vi "Main.vi"() -> ()   [LabVIEW 2025]
uses:
  Controls/Wheel_data.ctl
  Controls/Spork plot.ctl
  Controls/Spoke_stats.ctl
  Controls/Spork type.ctl
  Controls/Tension.ctl
  Controls/Tension_Output.ctl
  Controls/Runout.ctl
  Controls/Runout Output.ctl
  Controls/Nippel Turn Direction.ctl
  Controls/Aditional Info.ctl
  Controls/States.ctl
  <vilib>/Utility/NIReport.llb/NI_ReportGenerationCore.lvlib
panel:
  in  "Tab Control":enum32{"General", "Runout", "Tencion", "Export"}(tab)
  in  "Spokes":T1 {"Spokes crosses" min=0 max=4; "Spokes number" min=0 max=200 step=2}
  out "Wheel Visualation":cluster{dbl[], dbl[]}[](graph)
  in  "Stop":bool
  in  "Runout":bool
  out "Runout Graph":T3[](graph)
  out "Spork Measured":i32[](array[numeric])
  out "Runout Measurement":T4[](array[typedef])
  out "Runout Standard Diviation":dbl
  out "Runout Average":dbl
  in  "Spoke Tension Left":dbl[](array[numeric])
  in  "Variance":dbl min=0.0 max=25.0 step=5.0 format="%.0f %%"
  in  "Spoke Tension Right":dbl[](array[numeric])
  out "Tension Output Left":T6[](array[typedef])
  out "Tension Output Right":T6[](array[typedef])
  out "Spokes Tension":cluster{dbl[], dbl[]}[](graph)
  out "Average Tencion Right [kgf]":dbl
  out "Standard Diviation Right [kgf]":dbl
  out "Standard Diviation Left [kgf]":dbl
  out "Average Tencion Left [kgf]":dbl
  in  "Aditional Information":T7
  in  "Preview in Broweser":bool
  in  "Print":bool
  in  "Printer":u32(ring) items=["Default", "OneNote (Desktop) - Protected", "OneNote (Desktop)", "Microsoft Print to PDF"]
  in  "Wheel data":T8
  out "error out":errorcluster
  in  "error in":errorcluster
  # "Pass?"
  # "Pass?"
  # "Tension [kgf]"
  # "Tension [kgf]"
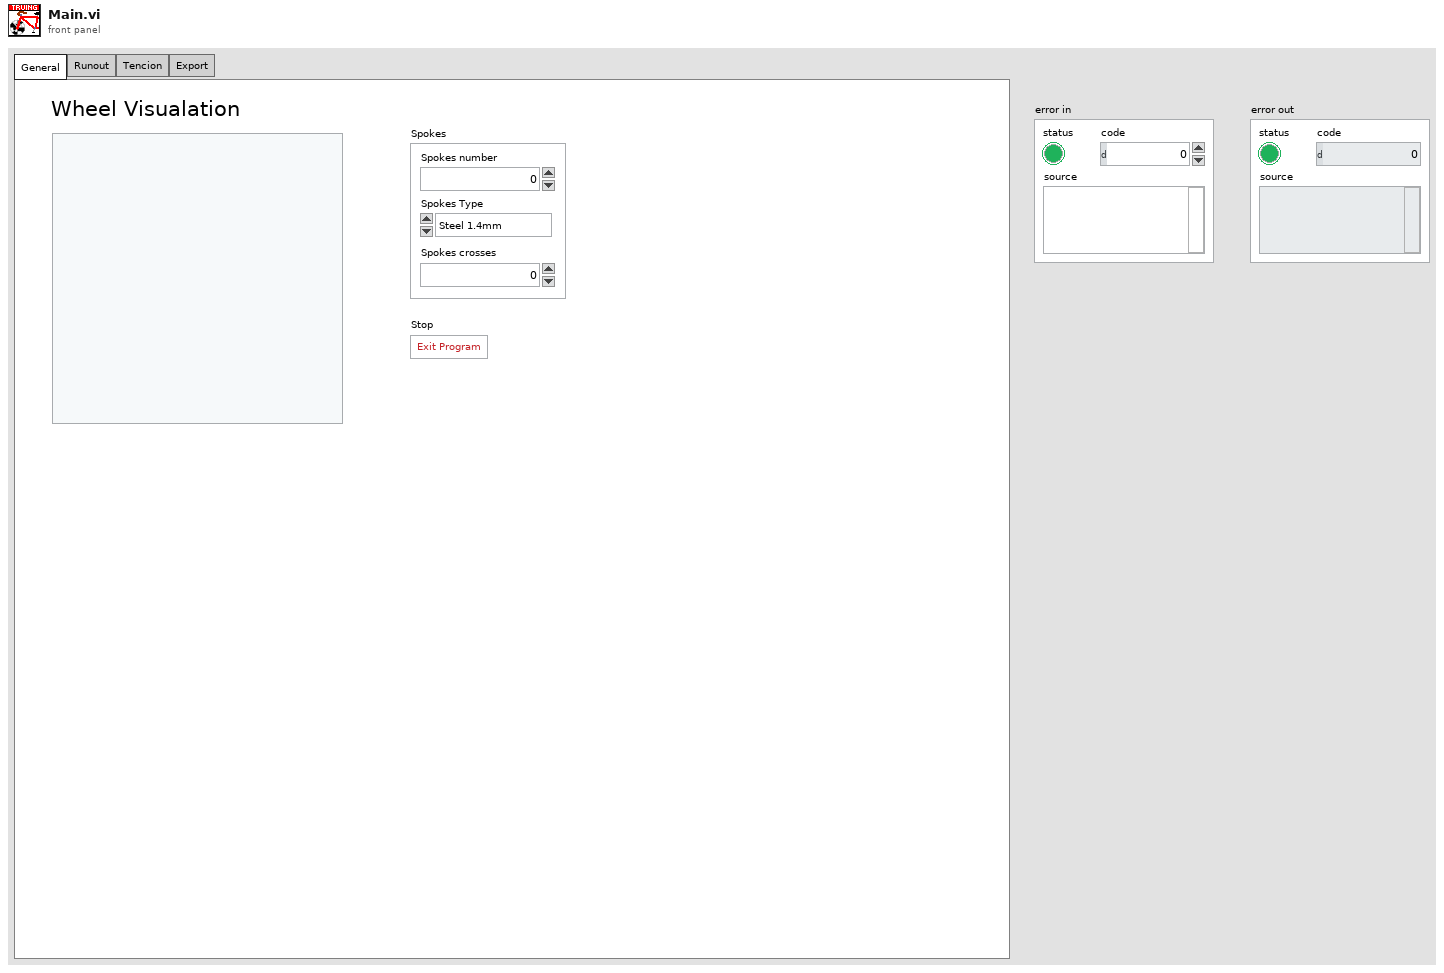
[diagram p1: front panel]
types:
  T1 = typedef "Spoke_stats.ctl" = cluster{"Spokes number":i32, "Spokes crosses":i32, "Spokes Type":T2}
  T2 = typedef "Spork type.ctl" = enum16{"Steel 1.4mm", "Steel 1.5mm", "Steel 1.6mm", "Steel 1.7mm", "Steel 1.8mm", "Steel 2mm", "Steel 2.3mm", "Steel 2.5mm", "Steel 2.6mm", "Aluminum 2.28mm", "Aluminum 2.54mm", "Aluminum 2.8mm", "Aluminum 3.3mm"}
  T3 = typedef "Spork plot.ctl" = cluster{"X":dbl[], "Y":dbl[]}
  T4 = typedef "Runout Output.ctl" = cluster{"Value":dbl, "Nippel Direction":T5}
  T5 = typedef "Nippel Turn Direction.ctl" = u16
  T6 = typedef "Tension_Output.ctl" = cluster{"Tenction [kgf]":dbl, "Within Limit":bool}
  T7 = typedef "Aditional Info.ctl" = cluster{"Name":string, "Rims":string, "Hub":string, "Notes":string, "Spokes":string, "Type":enum32{"Item 0", "Item 1"}, "Mechanic's Name":string}
  T8 = typedef "Wheel_data.ctl" = cluster{"Wheel Grapth":T3[], "Spokes":T1, "Tension":T9, "Runout":T10, "Avaliable Printers":string[], "Aditional Info":T7}
  T9 = typedef "Tension.ctl" = cluster{"Spokes Tension Left":dbl[], "Tension Graph":T3[], "Average Left":dbl, "Variance":dbl, "Std Div Left":dbl, "Average Right":dbl, "Std Div Right":dbl, "Tension Output Left":T6[], "Tension Output Right":T6[], "Spokes Tension Right":dbl[]}
  T10 = typedef "Runout.ctl" = cluster{"Runout Output":T4[], "Runout Graph":T3[], "Average":dbl, "Std Div":dbl, "Spoke Measured":i32[]}
  T11 = typedef "States.ctl" = enum16{"Error", "Init", "Idle", "Draw Wheel", "Tension", "Runout", "Report", "Stop"}
  T12 = typedef "LVStringsAndValuesArrayTypeDef_U32.ctl" = cluster{"String":string, "Value":u32}[]
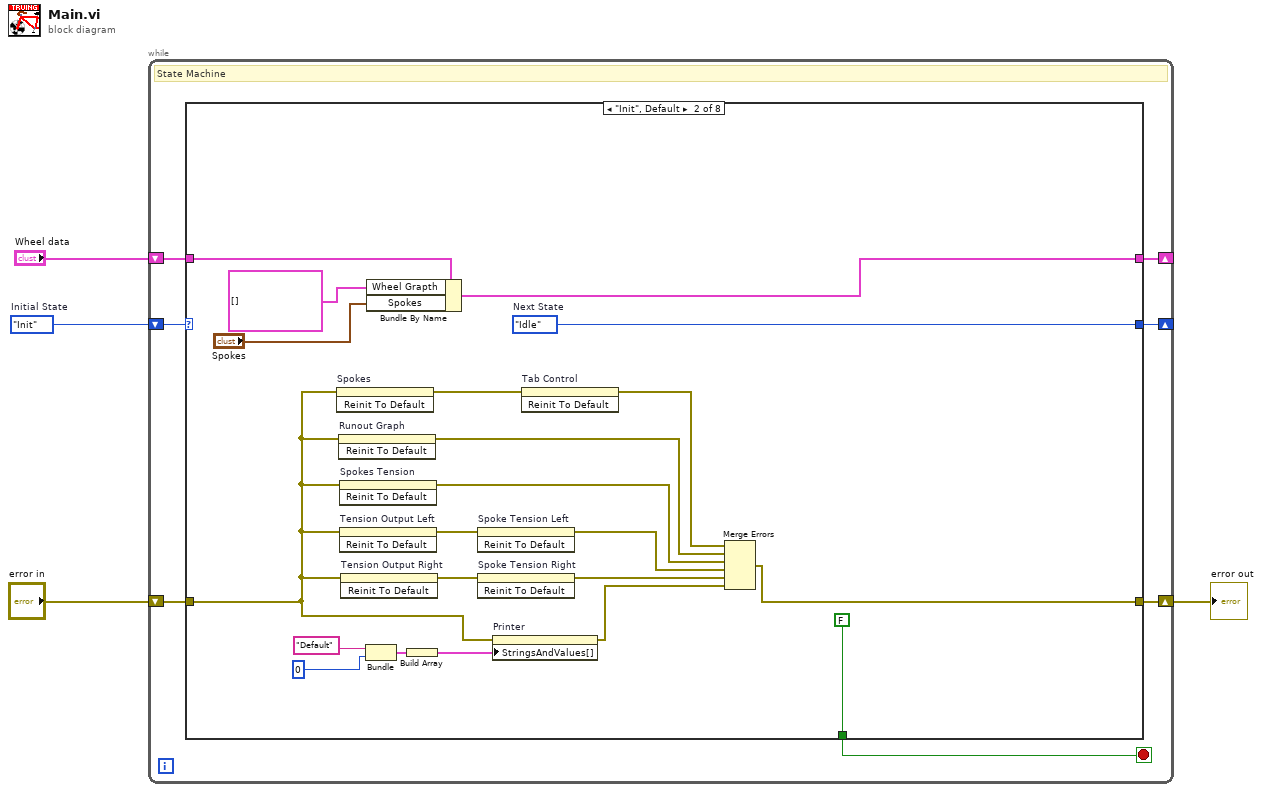
[diagram p0: block diagram]
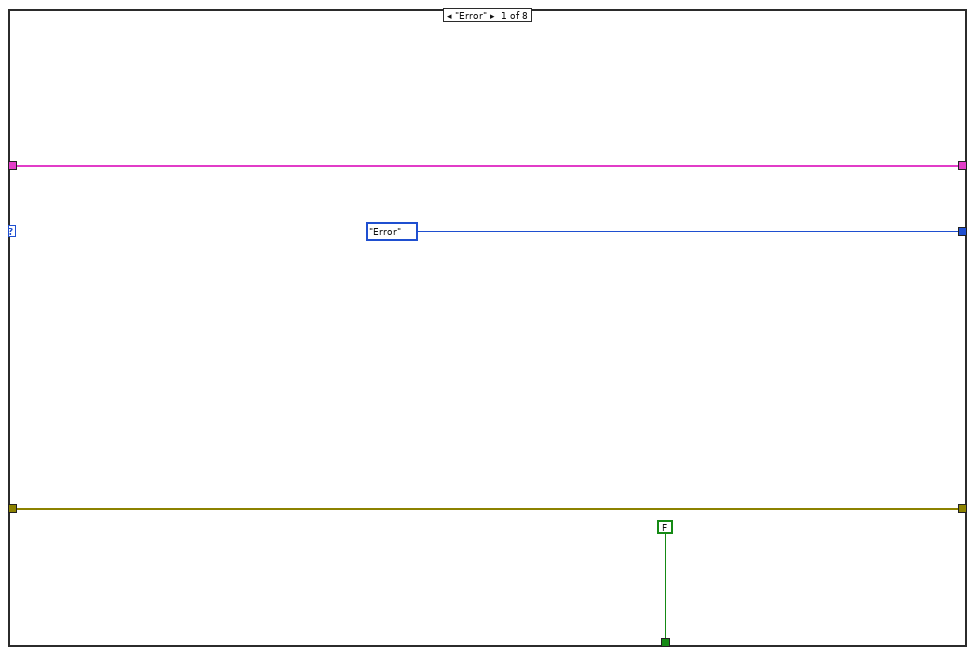
[diagram p2: hidden frame]
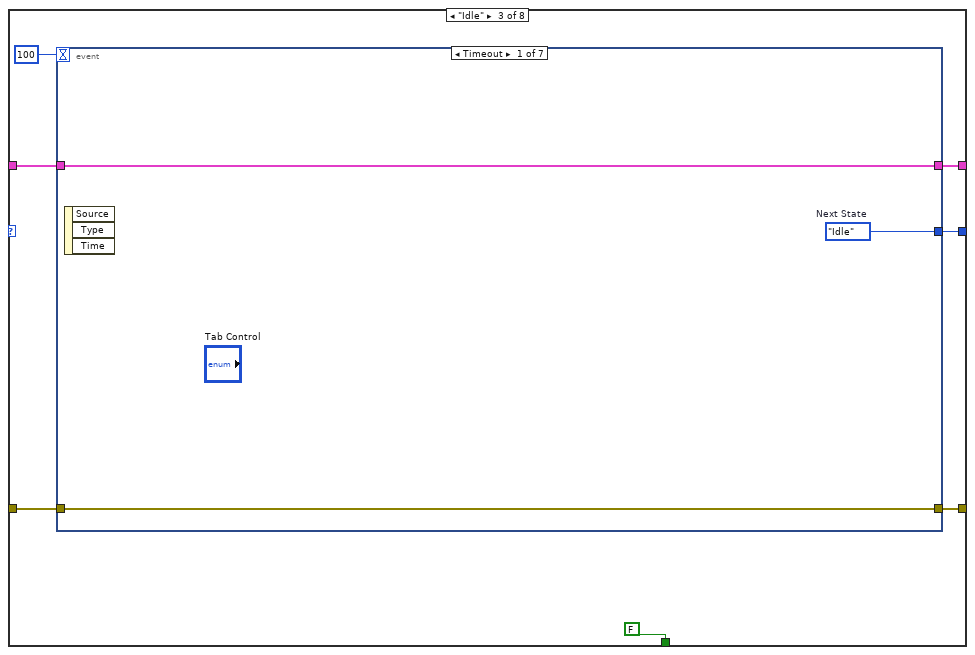
[diagram p3: hidden frame]
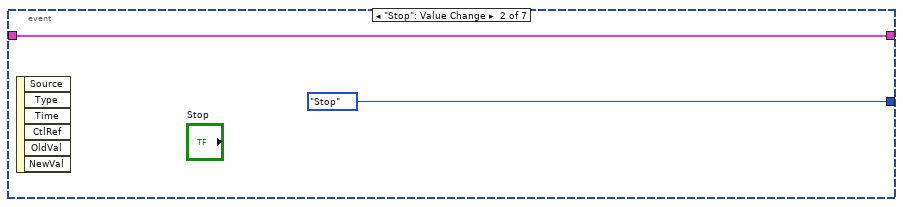
[diagram p4: hidden frame]
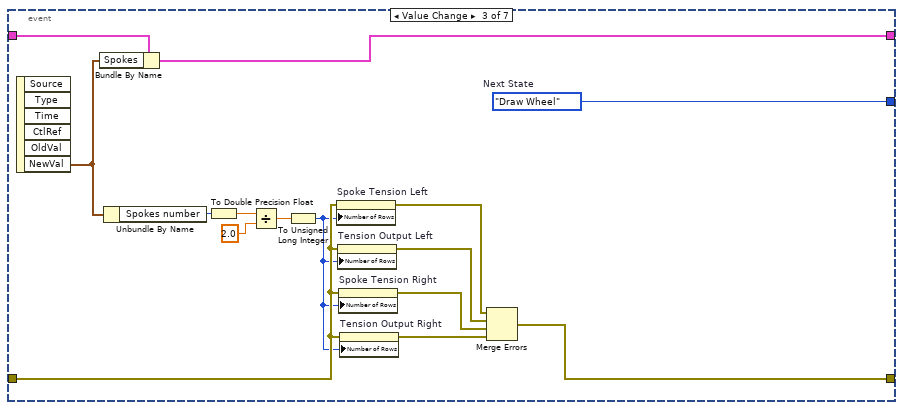
[diagram p5: hidden frame]
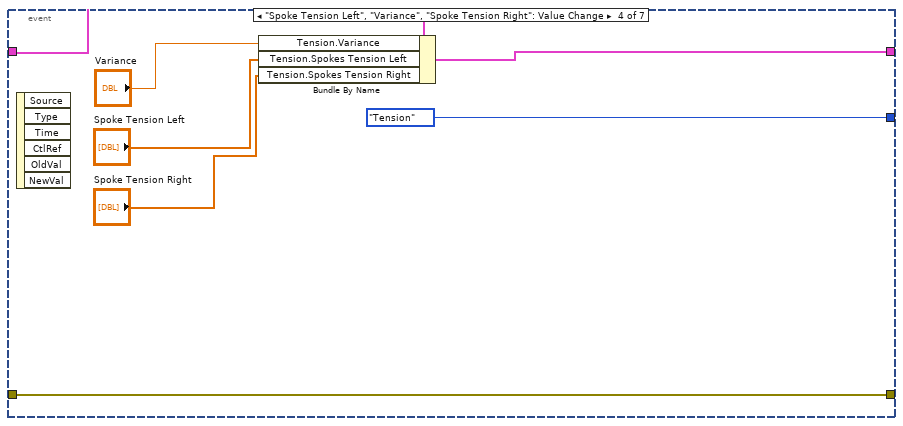
[diagram p6: hidden frame]
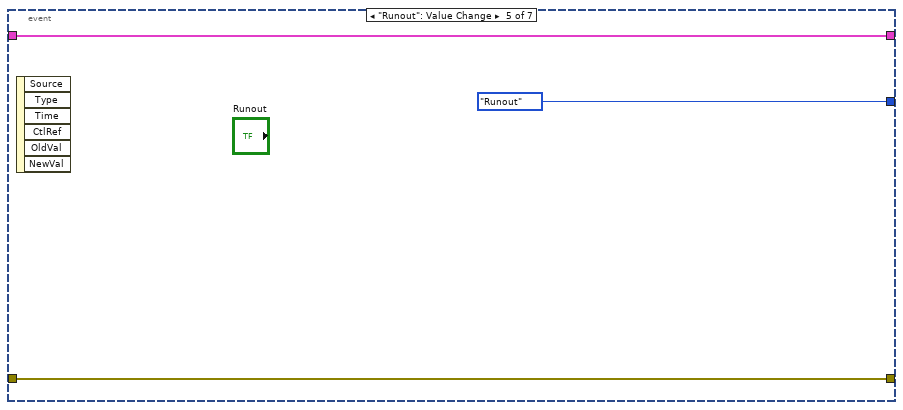
[diagram p7: hidden frame]
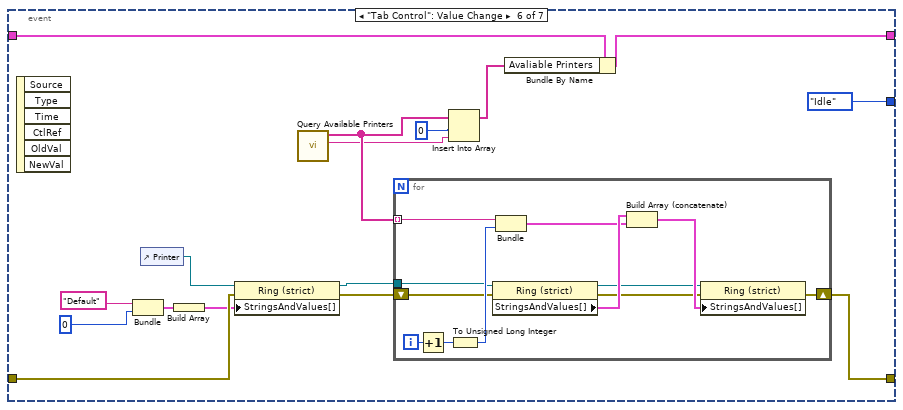
[diagram p8: hidden frame]
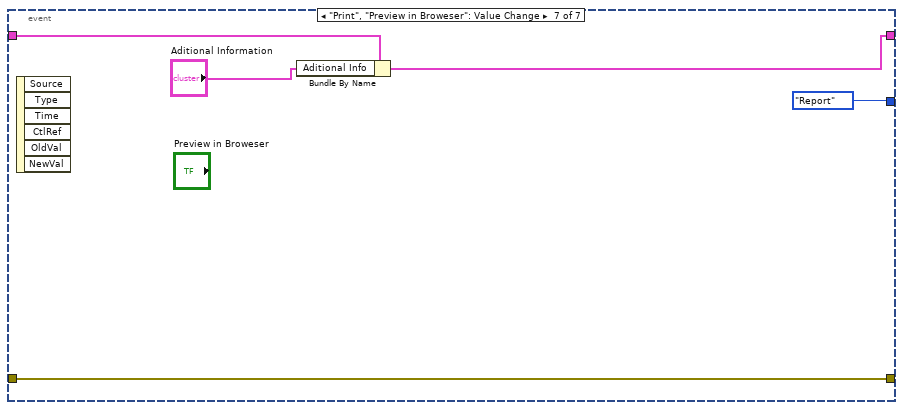
[diagram p9: hidden frame]
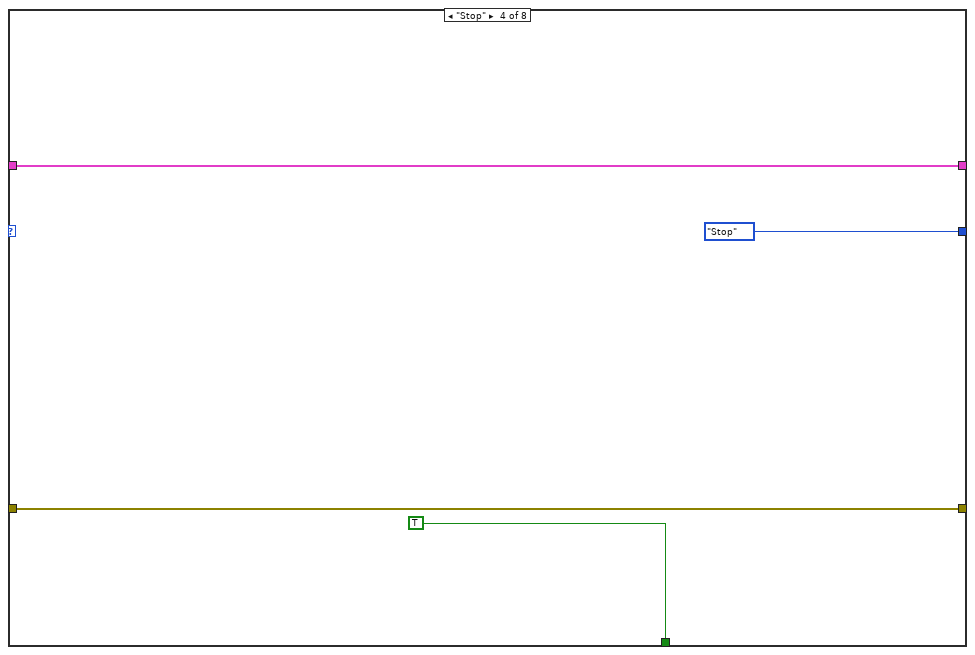
[diagram p10: hidden frame]
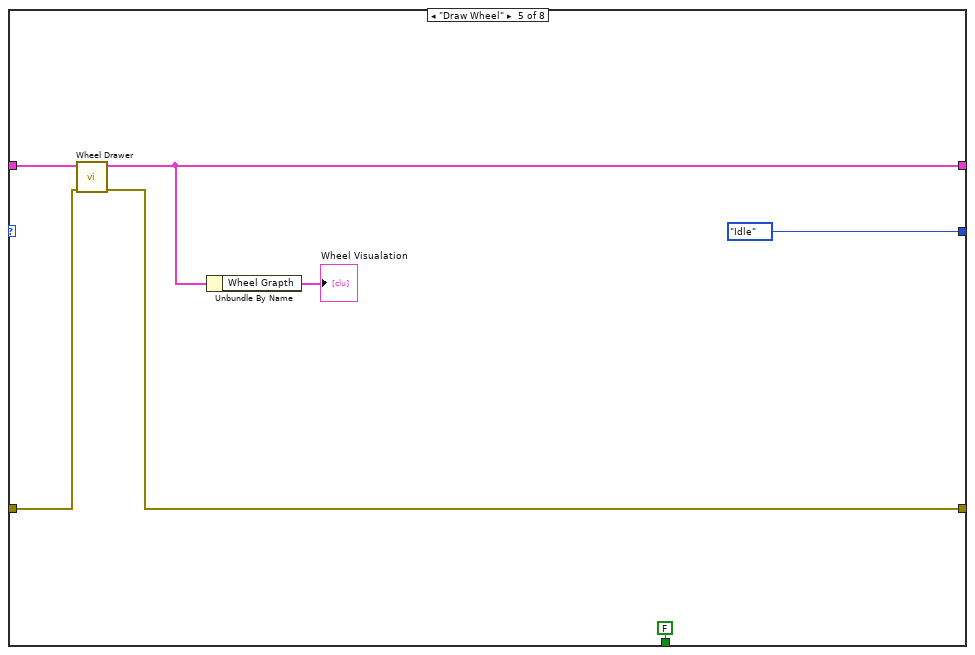
[diagram p11: hidden frame]
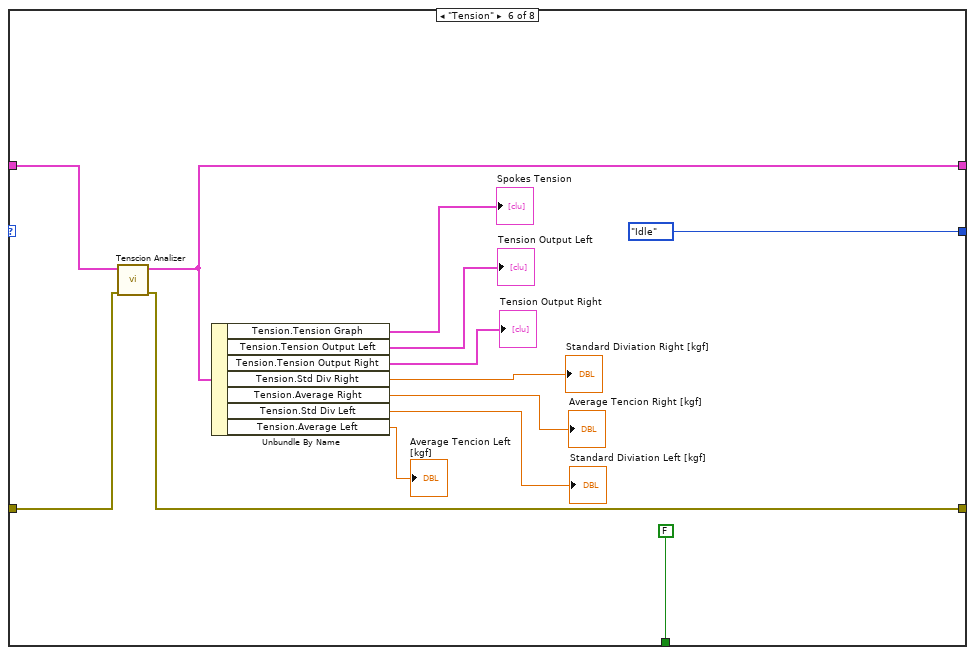
[diagram p12: hidden frame]
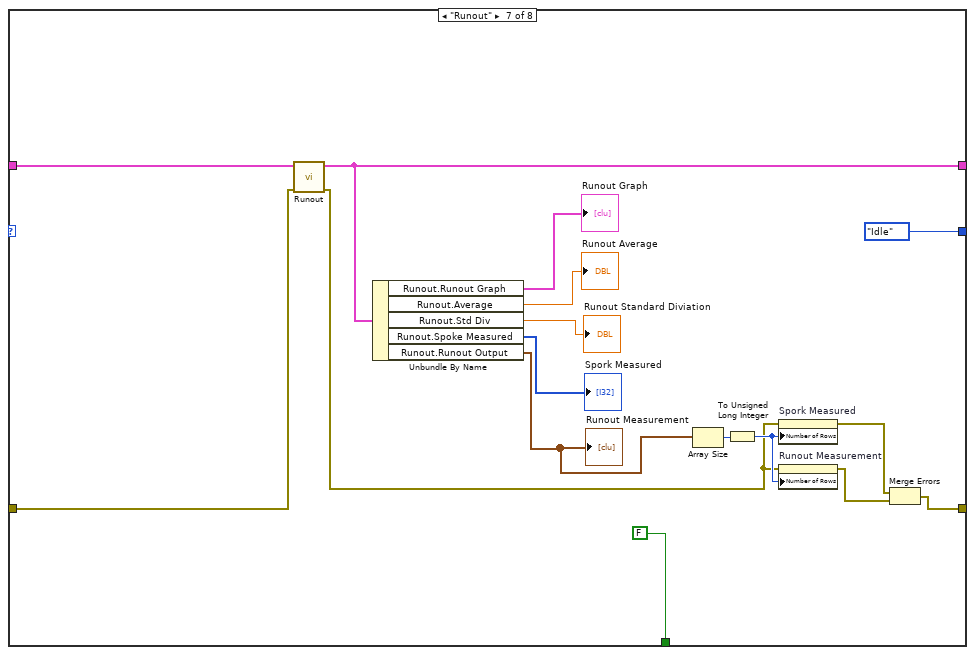
[diagram p13: hidden frame]
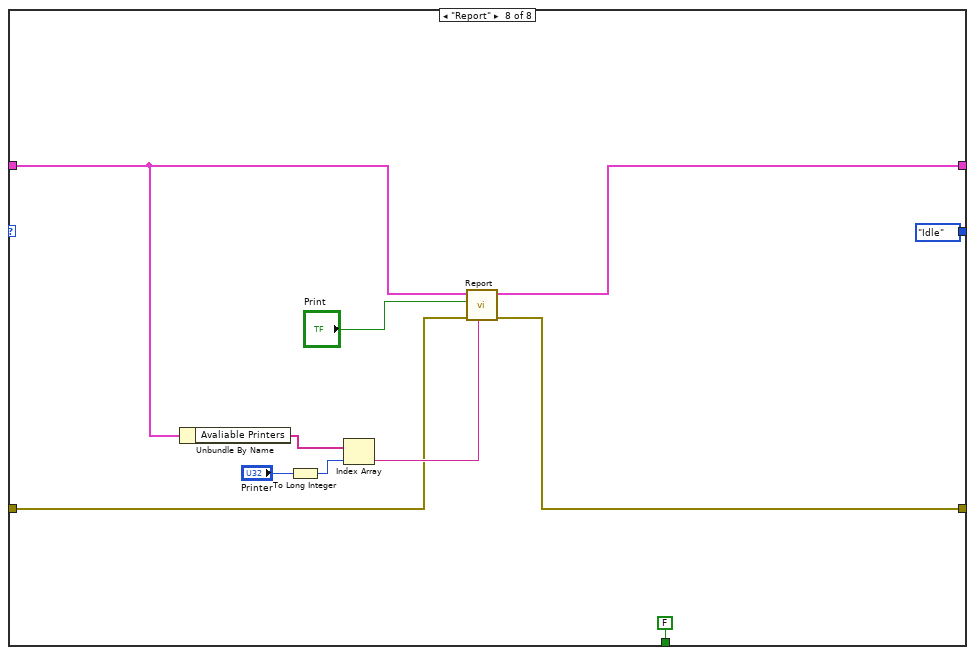
[diagram p14: hidden frame]
diagram:
  w4 = States."Init"  # Initial State
  n1 = while {
    shift-right: [w10] -> _
    shift-left: w4 -> [w11]
    shift-right: [w8] -> w2
    shift-left: "error in" -> [w9]
    shift-right: [w7] -> _
    shift-left: "Wheel data" -> [w6]
    stop <- w5 stop-if-true
    # "State Machine"
    n2 = case shown="\"Init\", Default" w11 {
      tunnel: [States."Error" ("Next State") w36 w37 States."Stop" ("Next State") States."Idle" ("Next State") States."Idle" ("Next State") States."Idle" ("Next State") States."Idle" ("Next State")] -> w10
      tunnel: w9 -> [w12 w18 w40 w110 w116 w123 w143 w151]
      tunnel: [w12 w28 w39 w110 w115 w122 w132 w150] -> w8
      tunnel: [w14 w35 w43 w108 w112 w124 w142 w149] -> w7
      tunnel: w6 -> [w14 w34 w42 w108 w117 w125 w144 w147]
      tunnel: [FALSE FALSE FALSE TRUE FALSE FALSE FALSE FALSE] -> w5
      frame "Error" {
      }
      frame "Init", Default {
        w36 = States."Idle"  # Next State
        n3 = invoke on="Spokes" class="Clust (strict)" method="Reinit To Default"(error in=w18) -> (error out=w17:errorcluster)  [unwired: 2 in, 2 out]
        n4 = invoke on="Runout Graph" class="XYGraph (strict)" method="Reinit To Default"(error in=w18) -> (error out=w30:errorcluster)  [unwired: 2 in, 2 out]
        n5 = invoke on="Spokes Tension" class="XYGraph (strict)" method="Reinit To Default"(error in=w18) -> (error out=w29:errorcluster)  [unwired: 2 in, 2 out]
        n6 = invoke on="Tension Output Left" class="Arr (strict)" method="Reinit To Default"(error in=w18) -> (error out=w27:errorcluster)  [unwired: 2 in, 2 out]
        n7 = invoke on="Tension Output Right" class="Arr (strict)" method="Reinit To Default"(error in=w18) -> (error out=w25:errorcluster)  [unwired: 2 in, 2 out]
        n8 = Bundle("Default", u32 0) -> (w21:cluster{string, u32})  [unwired: 1 in]
        n9 = Bundle By Name(cluster=w34, "Wheel Grapth"=T3[] [], "Spokes"="Spokes") -> (w35:T8)
        n10 = Build Array(w21) -> (w20:cluster{string, u32}[])
        n11 = invoke on="Spoke Tension Left" class="Arr (strict)" method="Reinit To Default"(error in=w27) -> (error out=w26:errorcluster)  [unwired: 2 in, 2 out]
        n12 = invoke on="Spoke Tension Right" class="Arr (strict)" method="Reinit To Default"(error in=w25) -> (error out=w24:errorcluster)  [unwired: 2 in, 2 out]
        n13 = property on="Printer" class="Ring (strict)"(error in=w18, "StringsAndValues[]"=w20) -> (error out=w19:errorcluster)  [unwired: 1 in, 1 out]
        n14 = invoke on="Tab Control" class="TabCtl (strict)" method="Reinit To Default"(error in=w17) -> (error out=w16:errorcluster)  [unwired: 2 in, 2 out]
        n15 = Merge Errors(w16, w30, w29, w26, w24, w19) -> (w28:errorcluster)
      }
      frame "Idle" {
        n16 = event shown="[0] Timeout" {
          selector: _ -> [_ _ _ _ _ _ _]
          dyn-events: _ -> [_ _ _ _ _ _ _]
          timeout: 100 -> [_ _ _ _ _ _ _]
          tunnel: [w44 w48 w61 w69 w73 w86 w103] -> w43
          tunnel: w42 -> [w44 w48 w63 w67 w73 w87 w104]
          tunnel: w40 -> [w45 _ w55 w70 w71 w77 w105]
          tunnel: [w45 _ w49 w70 w71 w89 w105] -> w39
          tunnel: [w46 States."Stop" ("Next State") w62 States."Tension" ("Enum") States."Runout" ("Enum") States."Idle" ("Enum") States."Report" ("Enum")] -> w37
          event Timeout {
            w46 = States."Idle"  # Next State
            n17 = event-data() -> ()  [unwired: 1 in, 3 out]
          }
          event "Stop": Value Change {
            n18 = event-data() -> ()  [unwired: 1 in, 6 out]
          }
          event Value Change {
            w62 = States."Draw Wheel"  # Next State
            n19 = event-data() -> ("NewVal"=w60:T1)  [unwired: 1 in, 5 out]
            n20 = Bundle By Name(cluster=w63, "Spokes"=w60) -> (w61:T8)
            n21 = Unbundle By Name(w60) -> ("Spokes number"=w59:i32)
            n22 = To Double Precision Float(number=w59) -> (double precision float=w58:dbl)
            n23 = Divide(x=w58, y=2.0) -> (x/y=w57:dbl)
            n24 = To Unsigned Long Integer(number=w57) -> (unsigned 32bit integer=w54:u32)
            n25 = property on="Spoke Tension Left" class="Arr (strict)"(error in=w55, "Number of Rows"=w54) -> (error out=w50:errorcluster)  [unwired: 1 in, 1 out]
            n26 = property on="Tension Output Left" class="Arr (strict)"(error in=w55, "Number of Rows"=w54) -> (error out=w51:errorcluster)  [unwired: 1 in, 1 out]
            n27 = property on="Spoke Tension Right" class="Arr (strict)"(error in=w55, "Number of Rows"=w54) -> (error out=w52:errorcluster)  [unwired: 1 in, 1 out]
            n28 = property on="Tension Output Right" class="Arr (strict)"(error in=w55, "Number of Rows"=w54) -> (error out=w53:errorcluster)  [unwired: 1 in, 1 out]
            n29 = Merge Errors(w50, w51, w52, w53) -> (w49:errorcluster)
          }
          event "Spoke Tension Left", "Variance", "Spoke Tension Right": Value Change {
            n30 = event-data() -> ()  [unwired: 1 in, 6 out]
            n31 = Bundle By Name(cluster=w67, "Tension.Variance"="Variance", "Tension.Spokes Tension Left"="Spoke Tension Left", "Tension.Spokes Tension Right"="Spoke Tension Right") -> (w69:T8)
          }
          event "Runout": Value Change {
            n32 = event-data() -> ()  [unwired: 1 in, 6 out]
          }
          event "Tab Control": Value Change {
            n33 = event-data() -> ()  [unwired: 1 in, 6 out]
            n34 = Bundle("Default", u32 0) -> (w79:cluster{string, u32})  [unwired: 1 in]
            n35 = control-ref of="Printer"() -> (w78:refnum<vi>)
            n36 = Build Array(w79) -> (w75:cluster{string, u32}[])
            n37 = property on="Property Node" class="Ring (strict)"(reference=w78, error in=w77, "StringsAndValues[]"=w75) -> (reference out=w74:refnum<vi>, error out=w76:errorcluster)
            n38 = call <vilib>:"Query Available Printers.vi"() -> ("default printer"=w84:string, "system configured printers"=w85:string[])  [unwired: 9 in, 1 out]
            n39 = for {
              tunnel: w85 -> [w96] mode=indexing
              shift-right: [w92] -> w89
              shift-left: w76 -> [w94]
              tunnel: w74 -> [w90]
              i -> [w101]
              n40 = Increment(x=w101) -> (x+1=w97:i32)
              n41 = To Unsigned Long Integer(number=w97) -> (unsigned 32bit integer=w98:u32)
              n42 = property on="Property Node" class="Ring (strict)"(reference=w90, error in=w94) -> (reference out=w91:refnum<vi>, error out=w93:errorcluster, "StringsAndValues[]"=w100:T12)
              n43 = Bundle("Printer Name"=w96, w98) -> (w95:cluster{"Printer Name":string, u32})  [unwired: 1 in]
              n44 = Build Array (concatenate)(w100, w95) -> (w99:T12)
              n45 = property on="Property Node" class="Ring (strict)"(reference=w91, error in=w93, "StringsAndValues[]"=w99) -> (error out=w92:errorcluster)  [unwired: 1 out]
            }
            n46 = Insert Into Array(array=w85, index=0, new element=w84) -> (w82:string[])
            n47 = Bundle By Name(cluster=w87, "Avaliable Printers"=w82) -> (w86:T8)
          }
          event "Print", "Preview in Broweser": Value Change {
            n48 = event-data() -> ()  [unwired: 1 in, 6 out]
            n49 = Bundle By Name(cluster=w104, "Aditional Info"="Aditional Information") -> (w103:T8)
          }
        }
      }
      frame "Stop" {
      }
      frame "Draw Wheel" {
        n50 = call "Wheel Drawer.vi"("error in"=w116, "Data In"=w117) -> ("error out"=w115:errorcluster, "Data Out"=w112:T8)  [unwired: 8 in]
        n51 = Unbundle By Name(w112) -> ("Wheel Grapth"=→"Wheel Visualation":T3[])
      }
      frame "Tension" {
        n52 = call "Tenscion Analizer.vi"("error in"=w123, "Data In"=w125) -> ("error out"=w122:errorcluster, "Data Out"=w124:T8)  [unwired: 8 in]
        n53 = Unbundle By Name(w124) -> ("Tension.Tension Graph"=→"Spokes Tension":T3[], "Tension.Tension Output Left"=→"Tension Output Left":T6[], "Tension.Tension Output Right"=→"Tension Output Right":T6[], "Tension.Std Div Right"=→"Standard Diviation Right [kgf]":dbl, "Tension.Average Right"=→"Average Tencion Right [kgf]":dbl, "Tension.Std Div Left"=→"Standard Diviation Left [kgf]":dbl, "Tension.Average Left"=→"Average Tencion Left [kgf]":dbl)
      }
      frame "Runout" {
        n54 = call "Runout.vi"("error in"=w143, "Data In"=w144) -> ("error out"=w135:errorcluster, "Data Out"=w142:T8)  [unwired: 8 in]
        n55 = Unbundle By Name(w142) -> ("Runout.Runout Graph"=→"Runout Graph":T3[], "Runout.Average"=→"Runout Average":dbl, "Runout.Std Div"=→"Runout Standard Diviation":dbl, "Runout.Spoke Measured"=→"Spork Measured":i32[], "Runout.Runout Output"=w131:T4[])
        "Runout Measurement" <- w131
        n56 = Array Size(array=w131) -> (size(s)=w137:i32)
        n57 = To Unsigned Long Integer(number=w137) -> (unsigned 32bit integer=w136:u32)
        n58 = property on="Spork Measured" class="Arr (strict)"(error in=w135, "Number of Rows"=w136) -> (error out=w134:errorcluster)  [unwired: 1 in, 1 out]
        n59 = property on="Runout Measurement" class="Arr (strict)"(error in=w135, "Number of Rows"=w136) -> (error out=w133:errorcluster)  [unwired: 1 in, 1 out]
        n60 = Merge Errors(w134, w133) -> (w132:errorcluster)
      }
      frame "Report" {
        n61 = Unbundle By Name(w147) -> ("Avaliable Printers"=w155:string[])
        n62 = To Long Integer(number="Printer") -> (32bit integer=w154:i32)
        n63 = Index Array(array=w155, index=w154) -> (element=w152:string)
        n64 = call "Report.vi"("Printer Name"=w152, "error in"=w151, "Print/Preview"="Print", "Data In"=w147) -> ("error out"=w150:errorcluster, "Data Out"=w149:T8)  [unwired: 6 in]
      }
    }
  }
  "error out" <- w2
